vi "Set Product Name.vi"(11 "Product Name":string="QC-X Thread Profiler") -> ()   [LabVIEW 2015, in "Tool Cfg.lvlib"]
uses:
  Tool Cfg.lvlib
  ConfigGLOB.vi
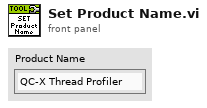
[diagram p1: front panel]
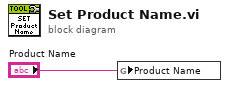
[diagram p0: block diagram]
diagram:
  n1 = global write "ConfigGLOB.vi" "Product Name"("Product Name") -> ()
